vi "OAT Orbit Locate Resampled Waveform Segment.vi"(8 "tach cycles":i32=1, 9 "orbit segment":cluster{"position":dbl, "tach duty":dbl} {"tach duty" format="%.2f"; "position" format="%.2f"}, 10 "pulse/revolution (1)":i32=1, 11 "speed profile":T1 {"speed [RPM]" format="%.2f"; "time [s]" format="%.2f"}) -> (1 "instant RPM":dbl format="%.2f", 2 "duration":dbl format="%.2f", 3 "start points":dbl[](array[numeric]) format="%.2f")   [LabVIEW 2017]
uses:
  <vilib>/addons/Sound and Vibration/Order Analysis/Tach Process/SubVIs/speed profile.ctl
  <vilib>/addons/Sound and Vibration/Order Analysis/Tach Process/SoundVib_TachProcess.lvlib
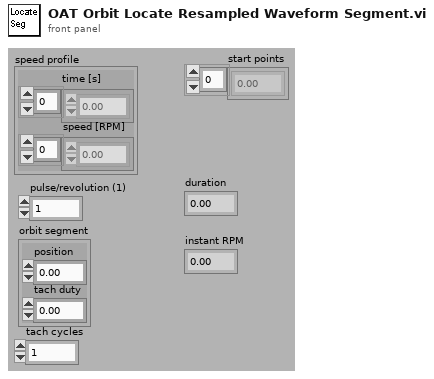
[diagram p1: front panel]
types:
  T1 = typedef "SoundVib_TachProcess.lvlib/speed profile.ctl" = cluster{"time [s]":dbl[], "speed [RPM]":dbl[]}
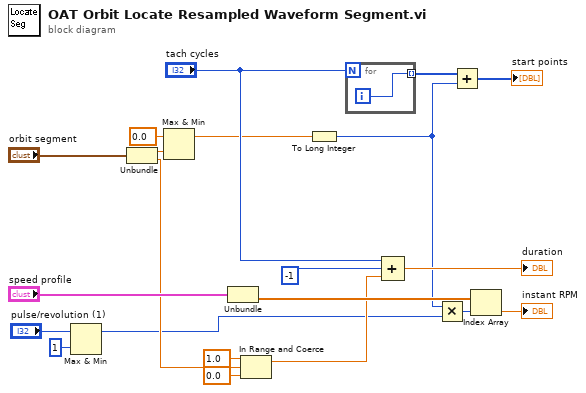
[diagram p0: block diagram]
diagram:
  n1 = Max & Min(x="pulse/revolution (1)", y=1) -> (max(x,y)=w2:i32)  [unwired: 1 out]
  n2 = Unbundle("orbit segment") -> ("position"=w16:dbl, "tach duty"=w5:dbl)
  n3 = Max & Min(x=0.0 ("y"), y=w16) -> (max(x,y)=w14:dbl)  [unwired: 1 out]
  n4 = Unbundle("speed profile") -> ("speed [RPM]"=w19:dbl[])  [unwired: 1 out]
  n5 = In Range and Coerce(upper limit=1.0, x=w5, lower limit=0.0) -> (coerced(x)=w4:dbl)  [unwired: 1 out]
  n6 = To Long Integer(number=w14) -> (32bit integer=w6:i32)
  n7 = for {
    N: "tach cycles" -> [_]
    tunnel: [w22] -> w18 mode=indexing
    i -> [w22]
  }
  n8 = Compound Arithmetic op=ADD("tach cycles", -1, w4) -> (→"duration":dbl)
  n9 = Multiply(x=w6, y=w2) -> (x*y=w20:i32)
  n10 = Add(x=w18, y=w6) -> (x+y=→"start points":i32[])
  n11 = Index Array(array=w19, index=w20) -> (element=→"instant RPM":dbl)
